vi "TargetLights.vi"(7 "DO Channels":u8[](array[numeric]), 8 "Error In":errorcluster, 9 "Hit?":bool, 10 "Target Number":u64=1 min=1 max=3, 11 "LINX Resource":T1) -> (0 "Error Out":errorcluster, 3 "LINX Resource 2":T1)   [LabVIEW 2022 SP3]
doc: "Setup Digital channels such that the order is:\n1 Ready\n1 Hit\n2 Ready\n2 Hit\n3 Ready\n3 Hit"
uses:
  <vilib>/MakerHub/LINX/Private/Type Defs/LINX Ref.ctl
  <vilib>/MakerHub/LINX/Private/Type Defs/Platform.ctl
  <vilib>/MakerHub/LINX/Private/Type Defs/Interface.ctl
  <vilib>/MakerHub/LINX/Private/Device/Type Defs/LINX Device Config.ctl
  <vilib>/MakerHub/LINX/Private/Device/Type Defs/TCP Config.ctl
  <vilib>/MakerHub/LINX/Private/Device/Type Defs/Channels.ctl
  <vilib>/MakerHub/LINX/Public/Peripherals/Digital/Digital Write N Chans.vi
  <vilib>/MakerHub/LINX/Private/Local IO/LinxDigitalWrite.vi
  <vilib>/MakerHub/LINX/Public/Utilities/Check Channel.vi
  <vilib>/MakerHub/LINX/Private/Utilties/Generate Error.vi
  <vilib>/MakerHub/LINX/LMH-LINX.lvlib
  <vilib>/MakerHub/LINX/Private/Device/Device.lvlib
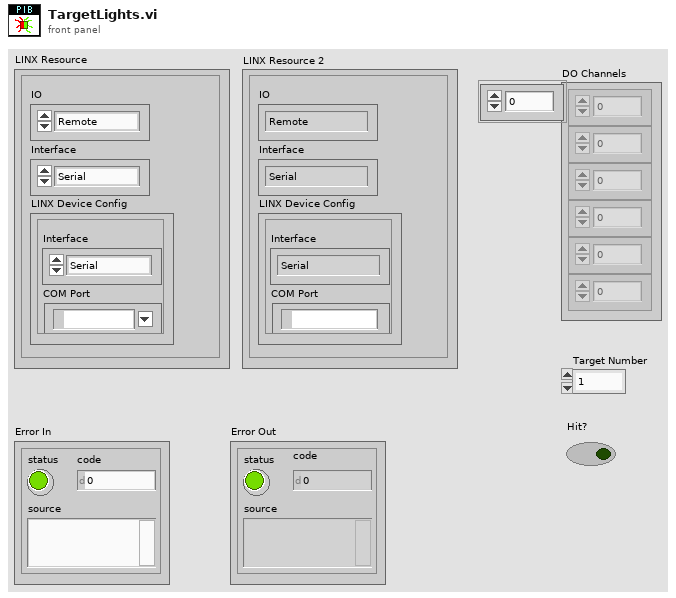
[diagram p1: front panel]
types:
  T1 = typedef "LMH-LINX.lvlib/LINX Ref.ctl" = cluster{"IO":T2, "Interface":T3, "LINX Device Config":T4}
  T2 = typedef "LMH-LINX.lvlib/Platform.ctl" = enum16{"Remote", "Local"}
  T3 = typedef "LMH-LINX.lvlib/Interface.ctl" = enum16{"Serial", "TCP"}
  T4 = typedef "LMH-LINX.lvlib/Device.lvlib/LINX Device Config.ctl" = cluster{"Interface":T3, "COM Port":refnum<visa-resource-name>, "TCP Configuration":T5, "Device Family":u8, "Device ID":u8, "Device Name":string, "TCP Ref":refnum<k5>, "Channels":T6}
  T5 = typedef "LMH-LINX.lvlib/Device.lvlib/TCP Config.ctl" = cluster{"IP Address":string, "Port":u16}
  T6 = typedef "LMH-LINX.lvlib/Channels.ctl" = cluster{"DI":u8[], "DO":u8[], "AI":u8[], "AO":u8[], "PWM":u8[], "QE":u8[], "UART":u8[], "I2C 2":u8[], "SPI":u8[], "CAN":u8[], "Servo":u8[], "AI Ref (V)":dbl, "AI Resolution (Bits)":u8, "AO Ref (V)":dbl, "AO Resolution (Bits)":u8}
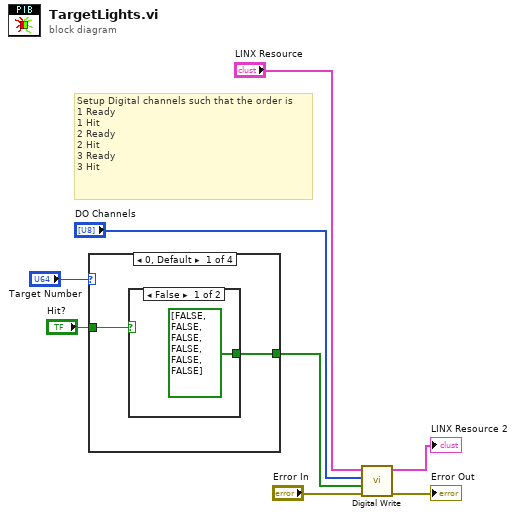
[diagram p0: block diagram]
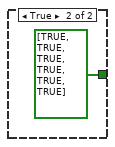
[diagram p2: hidden frame]
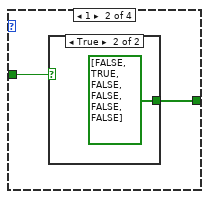
[diagram p3: hidden frame]
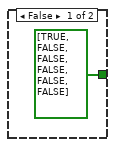
[diagram p4: hidden frame]
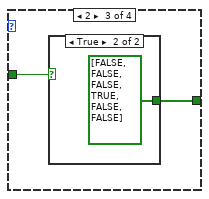
[diagram p5: hidden frame]
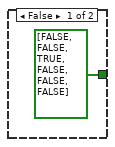
[diagram p6: hidden frame]
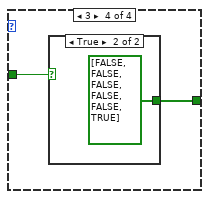
[diagram p7: hidden frame]
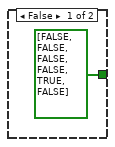
[diagram p8: hidden frame]
diagram:
  # "Setup Digital channels such that the order is \n1 Ready\n1 Hit\n2 Ready\n2 Hit\n3 Ready\n3 Hit"
  n1 = case shown="0, Default" "Target Number" {
    tunnel: "Hit?" -> [w9 w14 w18 w21]
    tunnel: [w10 w13 w17 w22] -> w1
    frame 0, Default {
      n2 = case shown="False" w9 {
        tunnel: [bool[] [FALSE, FALSE, FALSE, FALSE, FALSE, FALSE] bool[] [TRUE, TRUE, TRUE, TRUE, TRUE, TRUE]] -> w10
        frame False {
        }
        frame True {
        }
      }
    }
    frame 1 {
      n3 = case shown="True" w14 {
        tunnel: [bool[] [TRUE, FALSE, FALSE, FALSE, FALSE, FALSE] bool[] [FALSE, TRUE, FALSE, FALSE, FALSE, FALSE]] -> w13
        frame False {
        }
        frame True {
        }
      }
    }
    frame 2 {
      n4 = case shown="True" w18 {
        tunnel: [bool[] [FALSE, FALSE, TRUE, FALSE, FALSE, FALSE] bool[] [FALSE, FALSE, FALSE, TRUE, FALSE, FALSE]] -> w17
        frame False {
        }
        frame True {
        }
      }
    }
    frame 3 {
      n5 = case shown="True" w21 {
        tunnel: [bool[] [FALSE, FALSE, FALSE, FALSE, TRUE, FALSE] bool[] [FALSE, FALSE, FALSE, FALSE, FALSE, TRUE]] -> w22
        frame False {
        }
        frame True {
        }
      }
    }
  }
  n6 = call-poly <vilib>:"Digital Write.vi"("Error In"="Error In", "Values"=w1, "DO Channels"="DO Channels", "LINX Resource"="LINX Resource") -> ("Error Out"=→"Error Out":errorcluster, "LINX Resource"=→"LINX Resource 2":T1)  [unwired: 6 in]
